vi "Teleop.vi"(10 "Match Info":T1={"Autonomous Elapsed Seconds"=0.0, "TeleOp Elapsed Seconds"=0.0, "Disabled Elapsed Seconds"=0.0, "Visited Autonomous"=FALSE, "Visited TeleOp"=FALSE, "Visited Disabled"=FALSE, "Autonomous Settings"={"Autonomous Style"=enum."Independent", "VI Refnum"=refnum}}, 11 "Call Context":T2) -> ()   [LabVIEW 2018]
doc: "This VI is called for each TeleOp packet received from the DS where the robot is not disabled. It is often used to read from the joysticks and update I/O or to update setpoints for timed control loops. It should complete and return within 20 milliseconds or it may miss DS packets."
uses:
  <vilib>/Rock Robotics/WPI/DriverStation/WPI_DriverStationDerivedRobotMode.ctl
  <vilib>/Rock Robotics/WPI/DriverStation/WPI_DriverStationMatch Info.ctl
  <vilib>/Rock Robotics/WPI/Utilities/WPI_GetSetVariantRefNum.vi
  Robot Global Data.vi
  <vilib>/Rock Robotics/Network Tables/NT Write Boolean Array.vi
  <vilib>/Rock Robotics/Network Tables/NT Write Numeric Array.vi
  <vilib>/Rock Robotics/Network Tables/NT Read Boolean.vi
  <vilib>/Rock Robotics/Network Tables/NT Read Number.vi
panel:
  out "Sample Slider 0":dbl(slide) scale=0.0..5.0
  out "Sample Boolean 1":bool
  out "Sample Boolean 0":bool
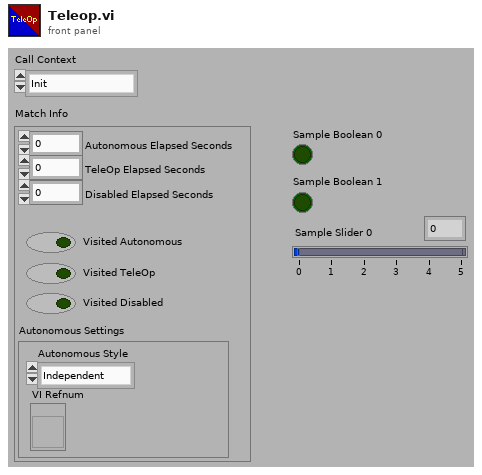
[diagram p1: front panel]
types:
  T1 = typedef "WPI_DriverStationMatch Info.ctl" = cluster{"Autonomous Elapsed Seconds":dbl, "TeleOp Elapsed Seconds":dbl, "Disabled Elapsed Seconds":dbl, "Visited Autonomous":bool, "Visited TeleOp":bool, "Visited Disabled":bool, "Autonomous Settings":cluster{"Autonomous Style":enum16{"Iterative", "Independent"}, "VI Refnum":refnum<vi>}}
  T2 = typedef "WPI_DriverStationDerivedRobotMode.ctl" = enum16{"Init", "Execute", "Stop"}
  T3 = enum16{"Idle", "Ground", "Hatch Low", "Hatch Mid", "Hatch High", "Cargo Low", "Cargo Mid", "Cargo High", "Cargo Ship", "Cargo Feed"}
  T4 = typedef "WPI_JoystickDevRef.ctl" = cluster{"Device":T5}
  T5 = typedef "WPI_JoystickDeviceEnum.ctl" = enum16{"USB 0", "USB 1", "USB 2", "USB 3", "USB 4", "USB 5"}
  T6 = typedef "WPI_RobotDriveDevRef.ctl" = cluster{"DevStatus":errorcluster, "Motors[]":T7[], "Square Inputs":bool, "Max Output":dbl}
  T7 = typedef "WPI_MotorControlDeviceRef.ctl" = cluster{"DeviceStatus":errorcluster, "Type":T8, "PWM":cluster{"PWM Channel":T9, "DeadBand":T10}, "CAN":cluster{"Device Number":u8, "SetOutput VI Ref":variant, "GetOutput VI Ref":variant, "Enable VI Ref":variant, "Disable VI Ref":variant, "Data":variant}, "Invert":bool, "DIO PWM":cluster{"PWM \"Enable\" Channel":T9, "DIOChannel":T11, "PWM Rate":dbl}}
  T8 = typedef "WPI_MotorControlType.ctl" = enum16{"PWM", "CAN", "DIO PWM"}
  T9 = typedef "FPGA_DIOPWMChannel.ctl" = enum8{"PWM 0", "PWM 1", "PWM 2", "PWM 3", "PWM 4", "PWM 5", "PWM 6", "PWM 7", "PWM 8", "PWM 9", "PWM MXP 0", "PWM MXP 1", "PWM MXP 2", "PWM MXP 3", "PWM MXP 4", "PWM MXP 5", "PWM MXP 6", "PWM MXP 7", "PWM MXP 8", "PWM MXP 9", "Invalid"}
  T10 = typedef "WPI_PWMDeadband.ctl" = cluster{"Name":string, "maxPositivePwm":i32, "minPositivePwm":i32, "centerPwm":i32, "maxNegativePwm":i32, "minNegativePwm":i32, "angularRange":u16}
  T11 = typedef "FPGA_DIOChannel.ctl" = enum8{"DIO 0", "DIO 1", "DIO 2", "DIO 3", "DIO 4", "DIO 5", "DIO 6", "DIO 7", "DIO 8", "DIO 9", "DIO MXP 0", "DIO MXP 1", "DIO MXP 2", "DIO MXP 3", "DIO MXP 4", "DIO MXP 5", "DIO MXP 6", "DIO MXP 7", "DIO MXP 8", "DIO MXP 9", "DIO MXP 10", "DIO MXP 11", "DIO MXP 12", "DIO MXP 13", "DIO MXP 14", "DIO MXP 15", "SPI Port CS1", "SPI Port CS2", "SPI Port CS3", "SPI Port MISO", "SPI Port MOSI", "Invalid"}
  T12 = cluster{"Axes[0]":dbl, "Axes[1]":dbl, "Axes[2]":dbl, "Axes[3]":dbl, "Axes[4]":dbl, "Axes[5]":dbl, "Axes[6]":dbl, "Axes[7]":dbl, "Axes[8]":dbl}
  T13 = cluster{"Buttons[0]":bool, "Buttons[1]":bool, "Buttons[2]":bool, "Buttons[3]":bool, "Buttons[4]":bool, "Buttons[5]":bool, "Buttons[6]":bool, "Buttons[7]":bool, "Buttons[8]":bool, "Buttons[9]":bool, "Buttons[10]":bool}
  T14 = cluster{"Buttons[0]":bool, "Buttons[1]":bool, "Buttons[2]":bool, "Buttons[3]":bool, "Buttons[4]":bool, "Buttons[5]":bool, "Buttons[6]":bool, "Buttons[7]":bool, "Buttons[8]":bool}
  T15 = typedef "ElevatorAndShift2.ctl" = cluster{"Drive Shift":bool, "Ground":bool, "Hatch Low":bool, "Hatch Mid":bool, "Hatch High":bool, "Cargo Low":bool, "Cargo Mid":bool, "Cargo High":bool, "Cargo Ship":bool, "Cargo Feed":bool}
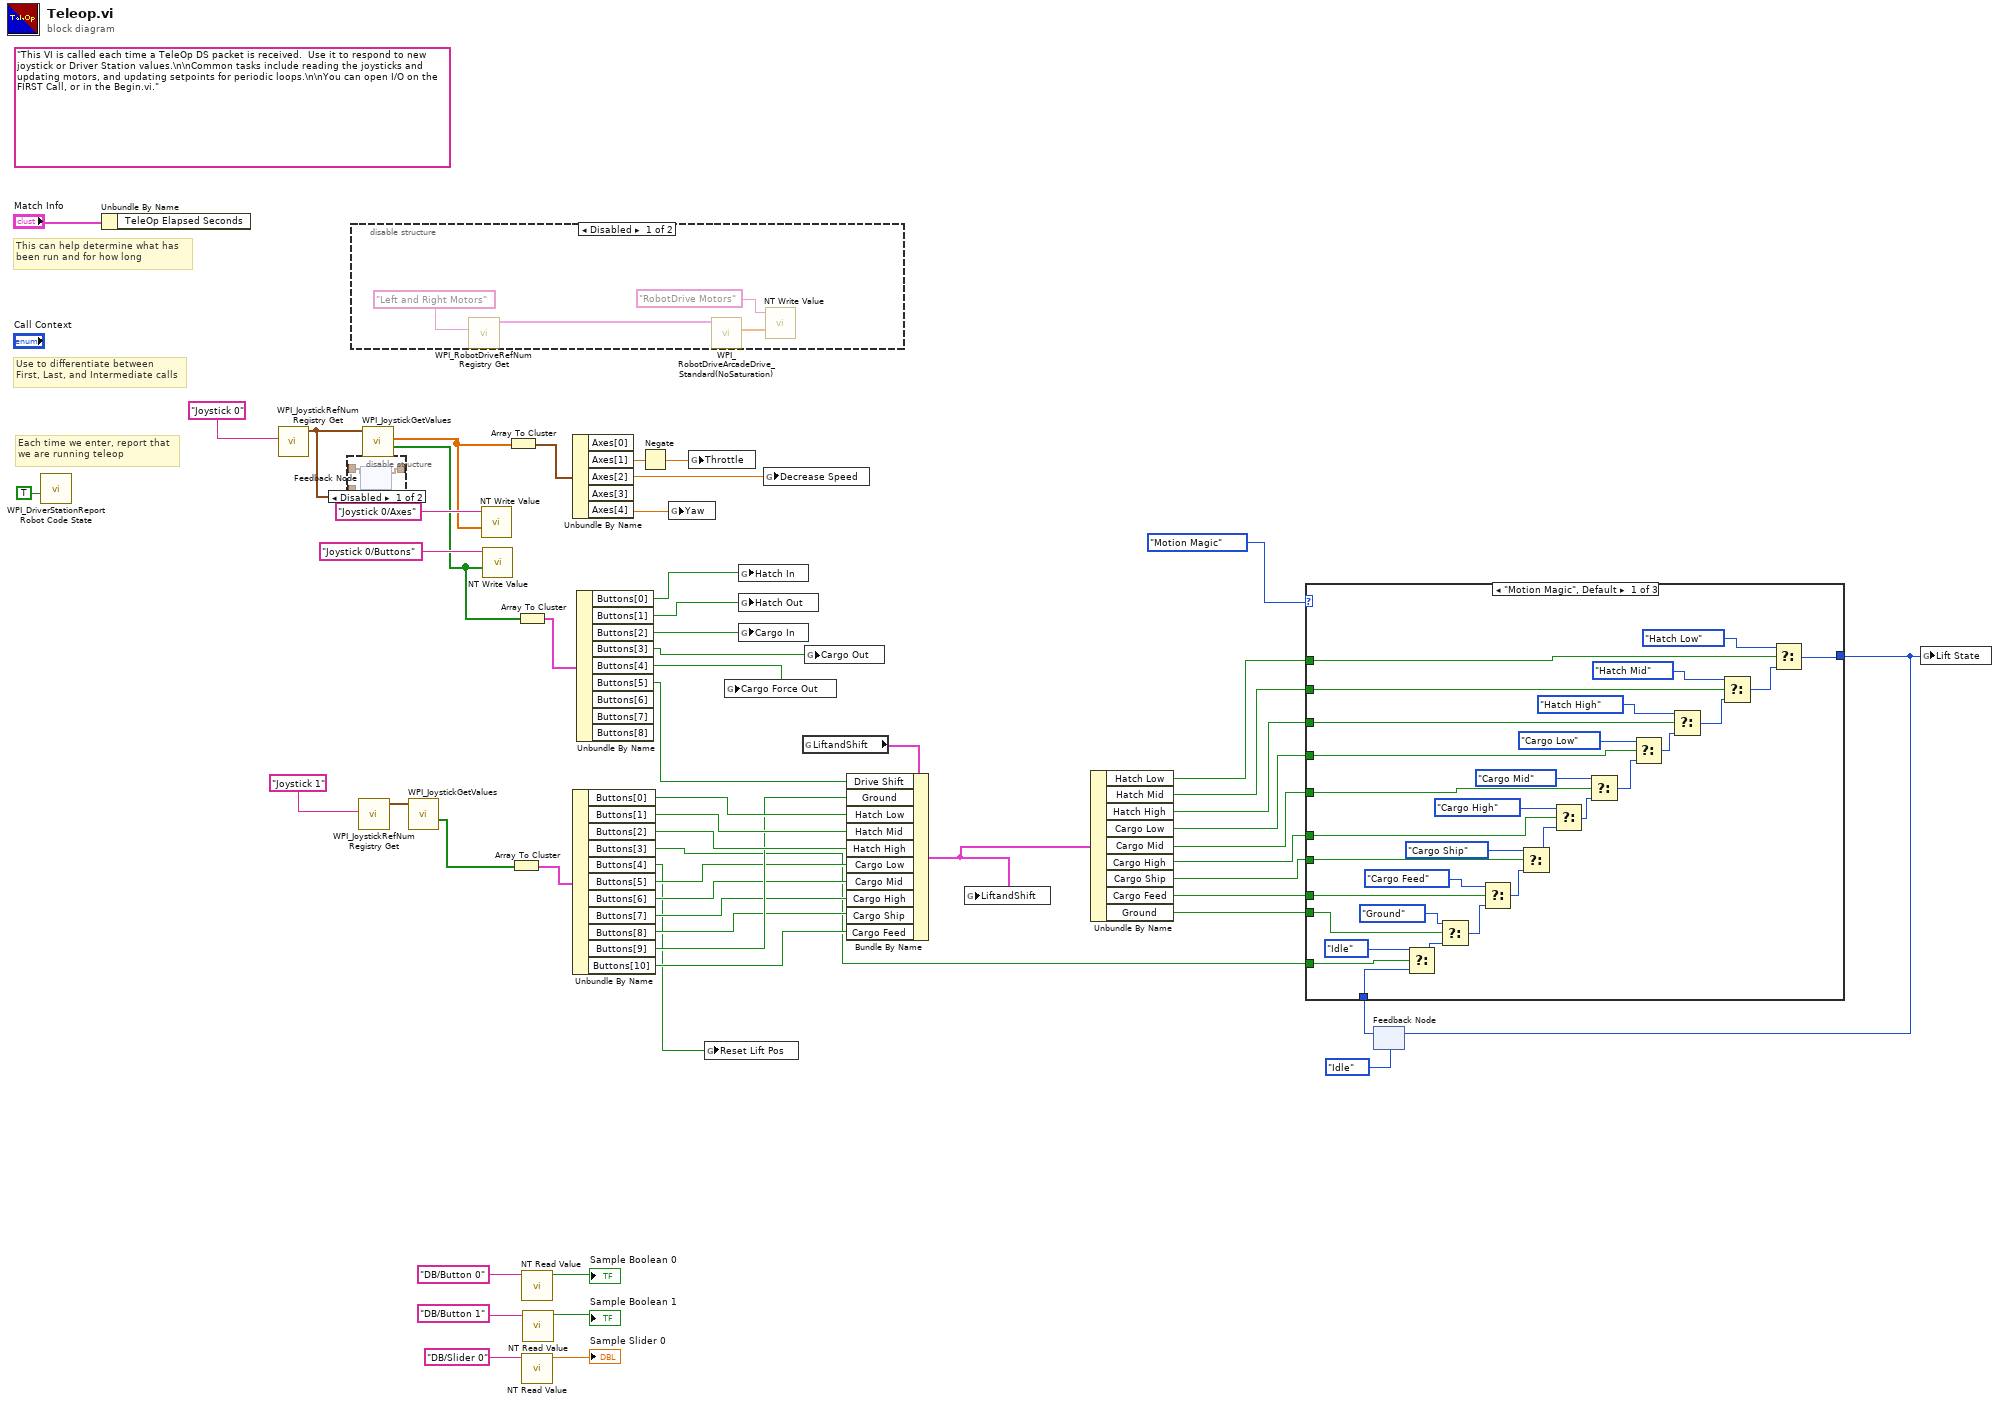
[diagram p0: block diagram]
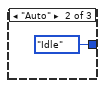
[diagram p2: hidden frame]
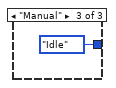
[diagram p3: hidden frame]
diagram:
  (unwired) "This VI is called each time a TeleOp DS packet is received.  Use it to respond to new joystick or Driver Station values.\n\nCommon tasks include reading the joysticks and updating motors, and updating setpoints for periodic loops.\n\nYou can open I/O on the FIRST Call, or in the Begin.vi."
  # "Each time we enter, report that\nwe are running teleop"
  # "Use to differentiate between\nFirst, Last, and Intermediate calls"
  # "This can help determine what has\nbeen run and for how long"
  n1 = call <vilib>:"WPI_DriverStationReport Robot Code State.vi"("TeleOp"=TRUE ("Autonomous")) -> ()  [unwired: 10 in, 1 out]
  n2 = Unbundle By Name("Match Info") -> ()  [unwired: 1 out]
  n3 = call <vilib>:"WPI_JoystickRefNum Registry Get.vi"("refnum name"="Joystick 0") -> ("JoystickDevRef"=w20:T4)  [unwired: 1 in, 9 out]
  n4 = disable-structure shown="Disabled" {
    disable-tunnel: _ -> [w59 _]
    disable-tunnel: [w58 _] -> _
    disable-tunnel: w20 -> [w57 _]
    frame Disabled {
      n5 = feedback #1(w57) -> (w58:T4)
      n6 = feedback-in #1(w59) -> ()
    }
    frame Enabled {
    }
  }
  n7 = disable-structure shown="Disabled" {
    frame Disabled {
      n8 = call <vilib>:"WPI_RobotDriveRefNum Registry Get.vi"("refnum name"="Left and Right Motors") -> ("RobotDriveDevRef"=w62:T6)  [unwired: 1 in, 9 out]
      n9 = call <vilib>:"WPI_RobotDriveArcadeDrive_Standard(NoSaturation).vi"("RobotDriveDevRef"=w62) -> ("Motor Values"=w60:dbl[])  [unwired: 3 in, 7 out]
      n10 = call-poly <vilib>:"NT Write Value.vi"("Numeric Array"=w60, "Name"="RobotDrive Motors") -> ()  [unwired: 9 in, 1 out]
    }
    frame Enabled {
    }
  }
  n11 = call <vilib>:"WPI_JoystickRefNum Registry Get.vi"("refnum name"="Joystick 1") -> ("JoystickDevRef"=w39:T4)  [unwired: 1 in, 9 out]
  n12 = call <vilib>:"WPI_JoystickGetValues.vi"("JoystickDevRef"=w20) -> ("Buttons"=w43:bool[], "Axes"=w45:dbl[])  [unwired: 6 in, 3 out]
  n13 = call <vilib>:"WPI_JoystickGetValues.vi"("JoystickDevRef"=w39) -> ("Buttons"=w40:bool[])  [unwired: 6 in, 4 out]
  n14 = call-poly <vilib>:"NT Write Value.vi"("Numeric Array"=w45, "Name"="Joystick 0/Axes") -> ()  [unwired: 9 in, 1 out]
  n15 = call-poly <vilib>:"NT Write Value.vi"("Boolean Array"=w43, "Name"="Joystick 0/Buttons") -> ()  [unwired: 9 in, 1 out]
  n16 = Array To Cluster(array=w45) -> (cluster=w44:T12)
  n17 = Array To Cluster(array=w40) -> (cluster=w41:T13)
  n18 = Array To Cluster(array=w43) -> (cluster=w42:T14)
  n19 = call-poly <vilib>:"NT Read Value.vi"("Name"="DB/Button 0" ("refnum name")) -> ("Boolean"=→"Sample Boolean 0":bool)  [unwired: 9 in, 1 out]
  n20 = call-poly <vilib>:"NT Read Value.vi"("Name"="DB/Slider 0" ("refnum name")) -> ("Numeric"=→"Sample Slider 0":dbl)  [unwired: 9 in, 1 out]
  n21 = call-poly <vilib>:"NT Read Value.vi"("Name"="DB/Button 1" ("refnum name")) -> ("Boolean"=→"Sample Boolean 1":bool)  [unwired: 9 in, 1 out]
  n22 = Unbundle By Name(w44) -> ("Axes[1]"=w22:dbl, "Axes[2]"=w6:dbl, "Axes[4]"=w23:dbl)  [unwired: 2 out]
  n23 = Unbundle By Name(w41) -> ("Buttons[0]"=w36:bool, "Buttons[1]"=w35:bool, "Buttons[2]"=w34:bool, "Buttons[3]"=w8:bool, "Buttons[4]"=w7:bool, "Buttons[5]"=w32:bool, "Buttons[6]"=w31:bool, "Buttons[7]"=w30:bool, "Buttons[8]"=w28:bool, "Buttons[9]"=w33:bool, "Buttons[10]"=w29:bool)
  n24 = Unbundle By Name(w42) -> ("Buttons[0]"=w26:bool, "Buttons[1]"=w25:bool, "Buttons[2]"=w27:bool, "Buttons[3]"=w1:bool, "Buttons[4]"=w2:bool, "Buttons[5]"=w19:bool)  [unwired: 3 out]
  n25 = Negate(x=w22) -> (-x=w21:dbl)
  n26 = global write "Robot Global Data.vi" "Yaw"(w23) -> ()
  n27 = global write "Robot Global Data.vi" "Throttle"(w21) -> ()
  n28 = global write "Robot Global Data.vi" "Reset Lift Pos"(w7) -> ()
  n29 = global write "Robot Global Data.vi" "Cargo Force Out"(w2) -> ()
  n30 = global write "Robot Global Data.vi" "Hatch In"(w26) -> ()
  n31 = global write "Robot Global Data.vi" "Hatch Out"(w25) -> ()
  n32 = global write "Robot Global Data.vi" "Cargo In"(w27) -> ()
  n33 = global write "Robot Global Data.vi" "Decrease Speed"(w6) -> ()
  n34 = global read "Robot Global Data.vi" "LiftandShift"() -> (w37:T15)
  n35 = global write "Robot Global Data.vi" "Cargo Out"(w1) -> ()
  n36 = Bundle By Name(cluster=w37, "Drive Shift"=w19, "Ground"=w33, "Hatch Low"=w36, "Hatch Mid"=w35, "Hatch High"=w34, "Cargo Low"=w32, "Cargo Mid"=w31, "Cargo High"=w30, "Cargo Ship"=w28, "Cargo Feed"=w29) -> (w24:T15)
  n37 = global write "Robot Global Data.vi" "LiftandShift"(w24) -> ()
  n38 = Unbundle By Name(w24) -> ("Hatch Low"=w10:bool, "Hatch Mid"=w11:bool, "Hatch High"=w12:bool, "Cargo Low"=w13:bool, "Cargo Mid"=w14:bool, "Cargo High"=w15:bool, "Cargo Ship"=w16:bool, "Cargo Feed"=w17:bool, "Ground"=w9:bool)
  n39 = feedback #2(T3."Idle" ("t")) -> (w5:T3)
  n40 = case shown="\"Motion Magic\", Default" enum16{"Motion Magic", "Auto", "Manual"}."Motion Magic" {
    tunnel: w17 -> [w93 _ _]
    tunnel: w16 -> [w90 _ _]
    tunnel: w15 -> [w87 _ _]
    tunnel: w14 -> [w84 _ _]
    tunnel: w13 -> [w81 _ _]
    tunnel: w12 -> [w79 _ _]
    tunnel: w11 -> [w74 _ _]
    tunnel: w10 -> [w73 _ _]
    tunnel: [w71 T3."Idle" ("t") T3."Idle" ("t")] -> w4
    tunnel: w9 -> [w69 _ _]
    tunnel: w8 -> [w65 _ _]
    tunnel: w5 -> [w64 _ _]
    frame "Motion Magic", Default {
      n41 = Select(t=T3."Idle", s=w65, f=w64) -> (s? t:f=w66:T3)
      n42 = Select(t=T3."Ground", s=w69, f=w66) -> (s? t:f=w68:T3)
      n43 = Select(t=T3."Cargo Feed", s=w93, f=w68) -> (s? t:f=w91:T3)
      n44 = Select(t=T3."Cargo Ship", s=w90, f=w91) -> (s? t:f=w88:T3)
      n45 = Select(t=T3."Cargo High", s=w87, f=w88) -> (s? t:f=w85:T3)
      n46 = Select(t=T3."Cargo Mid", s=w84, f=w85) -> (s? t:f=w82:T3)
      n47 = Select(t=T3."Cargo Low", s=w81, f=w82) -> (s? t:f=w78:T3)
      n48 = Select(t=T3."Hatch High", s=w79, f=w78) -> (s? t:f=w75:T3)
      n49 = Select(t=T3."Hatch Mid", s=w74, f=w75) -> (s? t:f=w72:T3)
      n50 = Select(t=T3."Hatch Low", s=w73, f=w72) -> (s? t:f=w71:T3)
    }
    frame "Auto" {
    }
    frame "Manual" {
    }
  }
  n51 = feedback-in #2(w4) -> ()
  n52 = global write "Robot Global Data.vi" "Lift State"(w4) -> ()
